vi "Launcher.vi"() -> ()   [LabVIEW 2014, in "HIJ File Viewer Demo App.lvlib"]
uses:
  HIJ File Viewer Demo App.lvlib
  HIJ File Viewer Demo App/HIJ File Viewer Demo App.lvclass
  <vilib>/ActorFramework/Actor/Actor.lvclass
panel:
  out "error out":errorcluster
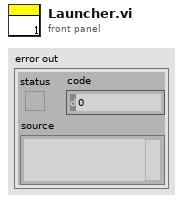
[diagram p1: front panel]
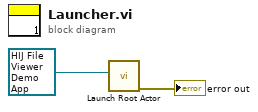
[diagram p0: block diagram]
diagram:
  n1 = call <vilib>:"Launch Root Actor.vi"("Actor"=refnum<class "HIJ File Viewer Demo App.lvclass"> refnum ("HIJ File Viewer Demo App.lvlib:HIJ File Viewer Demo App.lvclass")) -> ("error out"=→"error out":errorcluster)  [unwired: 9 in, 1 out]
